vi "simulate-robot-on-field.vi"() -> ()   [LabVIEW 2023]
uses:
  <vilib>/Rock Robotics/WPI/ThirdParty/JAS_Junk/TrajLib/TypeDef/FieldDisp_ElementPicture.ctl
  <vilib>/Rock Robotics/WPI/ThirdParty/JAS_Junk/TrajLib/VI/FieldDisp_Element_Rotate.vi
  <vilib>/Rock Robotics/WPI/ThirdParty/JAS_Junk/TrajLib/Conv_Meters_Inches.vi
  <vilib>/Rock Robotics/WPI/ThirdParty/JAS_Junk/TrajLib/Conv_Radians_Deg.vi
  SimulateDrive/SIM_Drive_Globals.vi
  <vilib>/picture/pixmap.llb/Flatten Pixmap.vi
  <vilib>/picture/pictutil.llb/Create Mask.vi
  <vilib>/picture/picture.llb/Draw Flattened Pixmap.vi
  <vilib>/Rock Robotics/WPI/ThirdParty/JAS_Junk/TrajLib/Trajectory_Library.lvlib
panel:
  out "ROBOT 2":T1
  out "Field Picture":picture
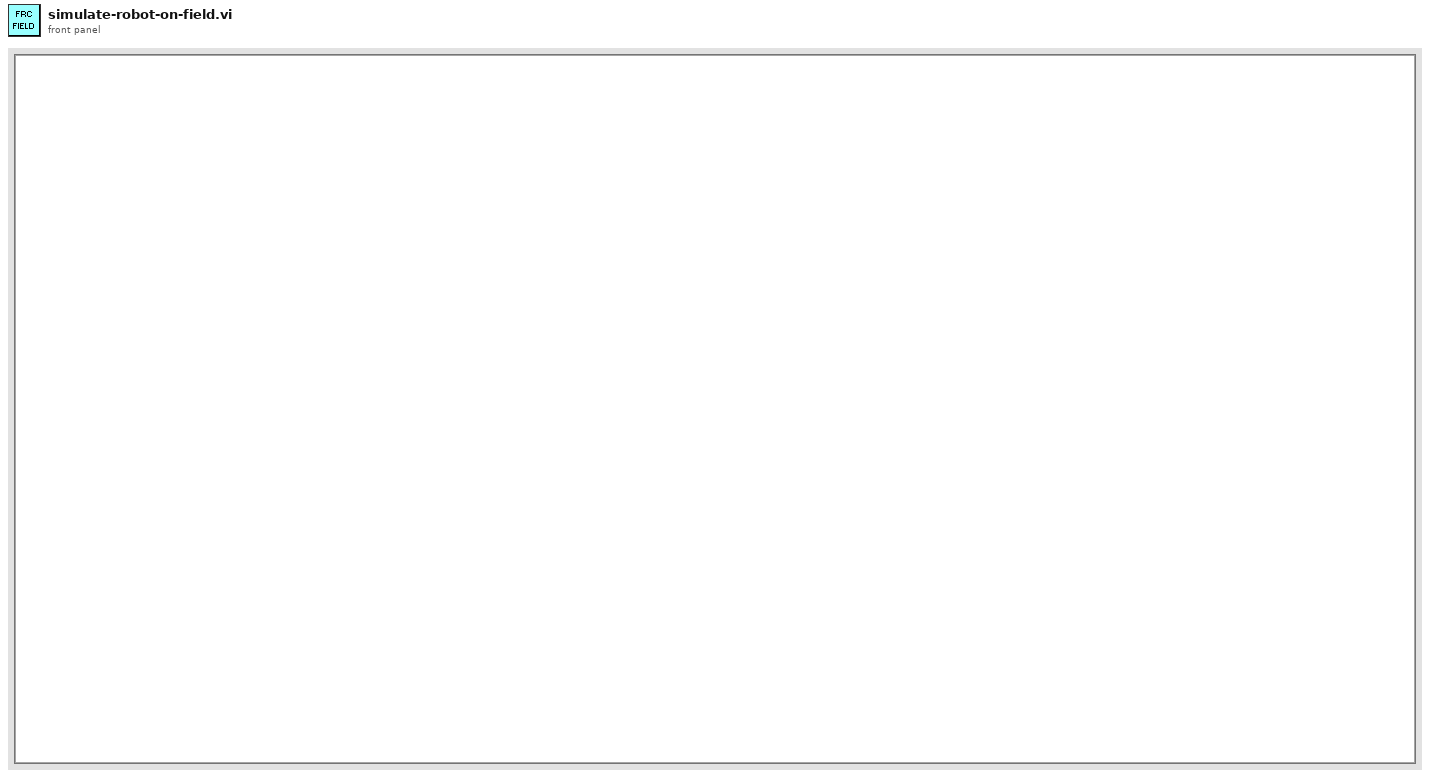
[diagram p1: front panel]
types:
  T1 = typedef "Trajectory_Library.lvlib/FieldDisp_ElementPicture.ctl" = picture
  T2 = typedef "Trajectory_Library.lvlib/FieldDisp_FieldElement.ctl" = cluster{"ONE-8-bit pixmap":u8[][], "Two-Array":cdb[][], "Three-Numeric":i32, "Four-Numeric":i32, "Five-Numeric":cdb, "Six-colors":u32[], "Seven-new element/subarray":u32, "Left Pixel":dbl, "Top Pixel":dbl, "Width Pix/Ft":dbl, "Height Pix/Ft":dbl, "Element Picture Ref":refnum<vi>}
  T3 = typedef "Trajectory_Library.lvlib/POSE2D.ctl" = cluster{"TRANSLATION":T4, "ROTATION":T5}
  T4 = typedef "Trajectory_Library.lvlib/TRANSLATION2D.ctl" = cluster{"X":dbl, "Y":dbl}
  T5 = typedef "Trajectory_Library.lvlib/ROTATION2D.ctl" = cluster{"VALUE":dbl, "COS":dbl, "SIN":dbl}
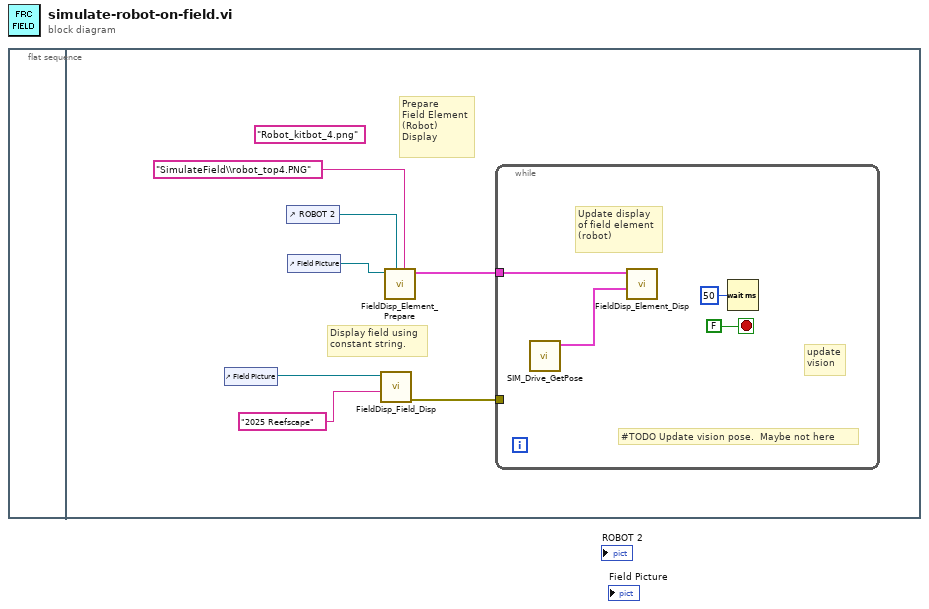
[diagram p0: block diagram]
diagram:
  n1 = flat-sequence {
    frame #0 {
    }
    frame #1 {
      (unwired) "Robot_kitbot_4.png" ("Picture FIle Name")
      # "Display field using\nconstant string."
      # "Prepare\nField Element\n(Robot)\nDisplay"
      n2 = control-ref of="Field Picture"() -> (w4:refnum<vi>)
      n3 = control-ref of="ROBOT 2"() -> (w6:refnum<vi>)
      n4 = control-ref of="Field Picture"() -> (w7:refnum<vi>)
      n5 = call <vilib>:"FieldDisp_Field_Disp.vi"("Field Selector"="2025 Reefscape", "Picture in"=w4) -> ("error out"=w3:errorcluster)  [unwired: 9 in]
      n6 = call <vilib>:"FieldDisp_Element_Prepare.vi"("Element File Name"="SimulateField\\robot_top4.PNG" ("name or relative path"), "Element Picture Ref"=w6, "Field Picture Ref"=w7) -> ("Field Element Info"=w5:T2)  [unwired: 7 in, 1 out]
      n7 = while {
        tunnel: w5 -> [w9]
        tunnel: w3 -> [_]
        stop <- FALSE stop-if-true
        # "#TODO Update vision pose.  Maybe not here"
        # "update\nvision"
        # "Update display\nof field element\n(robot)"
        n8 = call "SIM_Drive_GetPose.vi"() -> ("POSE"=w8:T3)  [unwired: 11 in]
        n9 = call <vilib>:"FieldDisp_Element_Disp.vi"("Element Pose"=w8, "Element Info"=w9) -> ()  [unwired: 10 in]
        n10 = Wait (ms)(milliseconds to wait=u32 50) -> ()  [unwired: 1 out]
      }
    }
  }
